vi "RP Test Template.vi"() -> ()   [LabVIEW 2024]
uses:
  RP Core/RP Communicator/RP Communicator.lvclass
  RP Status Offsets.ctl
panel:
  in  "bytes to read":i32=4
  out "Status response":u32=1 format="0x%x (%d)"
  out "bytes read":i32
  out "hex bytes":string
  in  "Send \"Connect client\"":bool=TRUE
  in  "Server address":string="192.168.1.100"
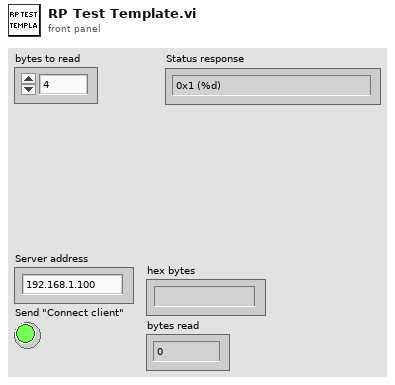
[diagram p1: front panel]
types:
  T1 = typedef "RP Status Offsets.ctl" = u16
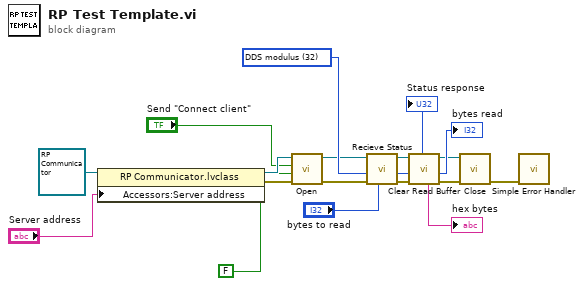
[diagram p0: block diagram]
diagram:
  w13 = T1 32 items=["Writer address"=0, "Record start position"=4, "Trig state and ID"=8, "Phase"=12, "X1"=16, "Y1"=20, "RxFIFO counter or  X2"=24, "TxFIFO counter or Y2"=28, "DDS modulus"=32] ("Status offsets")
  n1 = property class="RP Communicator.lvclass"(reference=refnum<class "RP Communicator.lvclass"> refnum ("RP Communicator.lvclass"), "Accessors:Server address"="Server address") -> (reference out=w16:refnum<class "RP Communicator.lvclass">, error out=w14:errorcluster)  [unwired: 1 in]
  n2 = call-dynamic "Open.vi"("error in (no error)"=w14, "Read config"=FALSE, "Send \"Connect client\""="Send \"Connect client\"", "RP Communicator in"=w16) -> ("error out"=w11:errorcluster, "RP Communicator out"=w12:refnum<class "RP Communicator.lvclass">)  [unwired: 6 in]
  n3 = call-dynamic "Recieve Status.vi"("bytes to read"="bytes to read", "error in (no error)"=w11, "Status offset"=w13, "RP Communicator in"=w12) -> ("error out"=w10:errorcluster, "Status response"=→"Status response":u32, "RP Communicator out"=w9:refnum<class "RP Communicator.lvclass">)  [unwired: 5 in]
  n4 = call-dynamic "Clear Read Buffer.vi"("error in (no error)"=w10, "RP Communicator in"=w9) -> ("error out"=w6:errorcluster, "bytes read"=→"bytes read":i32, "RP Communicator out"=w5:refnum<class "RP Communicator.lvclass">, "hex bytes"=→"hex bytes":string)  [unwired: 4 in, 2 out]
  n5 = call-dynamic "Close.vi"("error in (no error)"=w6, "RP Communicator in"=w5) -> ("error out"=w4:errorcluster)  [unwired: 8 in, 1 out]
  n6 = call <vilib>:"Simple Error Handler.vi"("error in (no error)"=w4) -> ()  [unwired: 4 in, 5 out]
